vi "Inverted Pendulum Simulation.vi"() -> ()   [LabVIEW 2018]
uses:
  <vilib>/Simulation/Scripting/Companion Diagram/SimConfigNode/SimParams.ctl
  <vilib>/Simulation/Scripting/Companion Diagram/SimConfigNode/_simSolvers.ctl
  <vilib>/Simulation/Implementation/Shared/SIMSCR Execution Mode.ctl
  <vilib>/Platform/TimedLoop/XDataNode/timing_clust.ctl
  <vilib>/Platform/TimedLoop/XDataNode/nitl_modes.ctl
  <vilib>/Platform/TimedLoop/XDataNode/wakeup.ctl
  <vilib>/Simulation/Param Hierarchy/Typedefs/SIMPH Param Control Actions.ctl
  <vilib>/Simulation/Implementation/Shared/NILVSim_ParamChanged.vi
  <vilib>/Simulation/Implementation/Shared/NILVSim_FinishedLate.vi
  <vilib>/Simulation/Implementation/Shared/NILVSIM_BeginStep.vi
  <vilib>/Simulation/DataSources/Implementation/NILVSim Signal Generator.llb/SIM Signal Generator (scalar).vi
  <vilib>/Simulation/SignalDisplay/Implementation/NILVSim Time Waveform.llb/SIM Time Waveform (scalar).vi
  <vilib>/Simulation/SignalArithmetic/Implementation/NILVSim Gain.llb/SIM Gain (scalar).vi
  <vilib>/Simulation/Utility/Implementation/SIM Halt.vi
  <vilib>/Simulation/ContinuousLinear/Implementation/NILVSim State Space.llb/SIM State Space Distributor (CD).vi
  <vilib>/Simulation/SignalArithmetic/Implementation/NILVSim Gain.llb/SIM Gain (vector,ScalarGain).vi
  <vilib>/Simulation/SignalDisplay/Implementation/NILVSim Time Waveform.llb/SIM Time Waveform (vector).vi
  <vilib>/Simulation/SignalArithmetic/Implementation/NILVSim Gain.llb/SIM Gain (vector,MatrixGain).vi
  <vilib>/Simulation/ContinuousLinear/Implementation/NILVSim State Space.llb/SIM State Space Collector (CD).vi
  <vilib>/Simulation/Implementation/Shared/NILVSim_Manager.vi
  <vilib>/Utility/error.llb/Clear Errors.vi
  <vilib>/Simulation/Implementation/Shared/NILVSim_FinalizeModel.vi
  <vilib>/imath/engines/lvmath2/RunTimeEngine/IndexRead/NIMS M(S,S).vi
  <instcachedir>/0/NIMS M(S,S)_AC51E74150A542F7991B9634C66F3096.lvgen/NIMS M(S,S)_AC51E74150A542F7991B9634C66F3096_000.vi
  <vilib>/imath/engines/lvmath2/RunTimeEngine/IndexRead/NIMS V(S).vi
  <instcachedir>/0/NIMS V(S)_0488751826AF41519A22953C041130DC.lvgen/NIMS V(S)_0488751826AF41519A22953C041130DC_000.vi
  <vilib>/imath/engines/lvmath2/RunTimeEngine/IndexReplace/NIMS M(S,S)=S.vi
  <instcachedir>/0/NIMS M(S,S)=S_5DAF17B45D8A4C8588C7CF468644990A.lvgen/NIMS M(S,S)=S_5DAF17B45D8A4C8588C7CF468644990A_000.vi
  <vilib>/imath/engines/lvmath2/RunTimeEngine/ErrorHandling/NIMS_Create Error From Enums.vi
  <vilib>/imath/engines/lvmath/Plug In/Control Design/BuiltInFunctions/ss/NIMS_CD_ss(A,B,C,D).vi
  <vilib>/imath/engines/lvmath2/RunTimeEngine/NodeEndStatement/NIMS_NodeEndStatement_Output.vi
  <instcachedir>/0/NIMS_NodeEndStatement_Output_53EC0D466D134D7ABD903AC30B43404B.lvgen/NIMS_NodeEndStatement_Output_53EC0D466D134D7ABD903AC30B43404B_011.vi
  <vilib>/imath/engines/lvmath2/RunTimeEngine/ErrorHandling/NIMS_Finalize Error.vi
  <vilib>/Simulation/Implementation/Shared/SIM Unbundle Sim Info.vi
  <vilib>/Simulation/Implementation/Shared/SIMSH Read Queue.vi
  <vilib>/Simulation/Implementation/Shared/NILVSim_Initialize.vi
  <vilib>/Simulation/Utility/Implementation/NILVSim Get Time and IsAcceptedStep.vi
  <vilib>/Simulation/Implementation/Shared/NILVSim_GetModelError.vi
  <vilib>/Simulation/Implementation/Shared/SIM Bundle Sim Info.vi
  <vilib>/Simulation/Scripting/Companion Diagram/SimConfigNode/SimDog.xnode
  <vilib>/addons/Control Design/_Model Construction/Model Typedefs.llb/CD State Space Model (MIMO).ctl
  <vilib>/addons/Control Design/_Model Construction/Model Typedefs.llb/CD General Elements.ctl
  <vilib>/Platform/TimedLoop/XDataNode/XDataNode.xnode
  <vilib>/Simulation/Implementation/XNodeFramework/SimXNode/SimX.xnode
  <vilib>/addons/Control Design/_Model Construction/NI_LinSys_Model Typedefs.lvlib
  <vilib>/Simulation/ContinuousLinear/Implementation/NILVSim State Space.llb/SIM State Space (CD).vi
  <vilib>/Platform/TimedLoop/XDataNode/XDNodeRunTimeDep.lvlib
  <vilib>/Simulation/Implementation/Shared/NI_SIM_Implementation.lvlib
panel:
  out "Reference":waveform(dbl)(graph)
  in  "Feedback Gain":dbl[][](array[numeric])
  out "Output":waveform(dbl)[](graph)=[{"t0"=timestamp(14.86 s since 1904-01-01), "dt"=1.0, "Y"=[20.0]}, {"t0"=timestamp(14.86 s since 1904-01-01), "dt"=1.0, "Y"=[19.893873916201358]}]
  out "State":waveform(dbl)[](graph)=[{"t0"=timestamp(14.86 s since 1904-01-01), "dt"=1.0, "Y"=[20.0]}, {"t0"=timestamp(14.86 s since 1904-01-01), "dt"=1.0, "Y"=[19.893873916201358]}]
  in  "Frequency (Hz)":dbl(slide)=0.2 min=0.0 max=0.5 step=0.05 scale=0.0..0.5 scale format="%#_3f"
  in  "Amplitude (deg)":dbl(slide)=20.0 min=0.0 max=40.0 step=5.0 scale=0.0..40.0
  in  "stop":bool
  # "Rotary Arm Reference Signal"
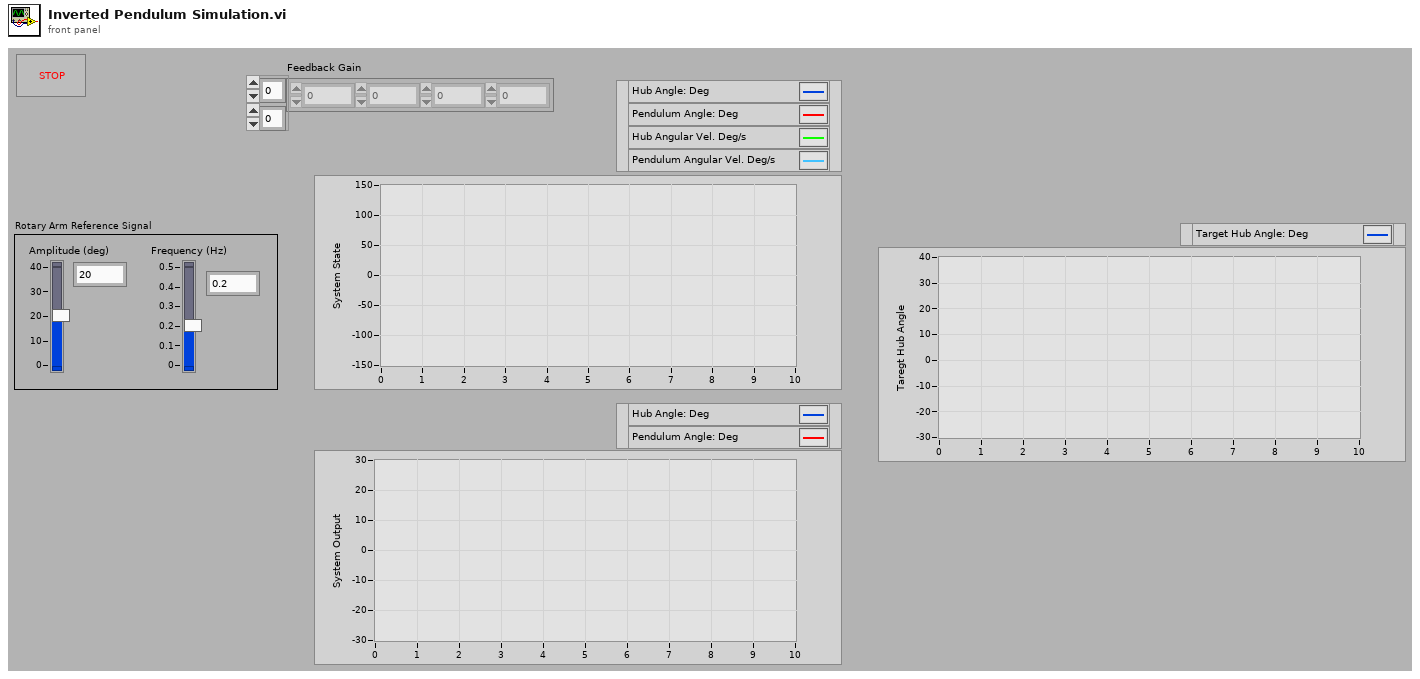
[diagram p1: front panel]
types:
  T1 = typedef "NI_LinSys_Model Typedefs.lvlib/CD State Space Model (MIMO).ctl" = cluster{"properties":T2, "A":dbl[][], "B":dbl[][], "C":dbl[][], "D":dbl[][], "StateNames":string[], "Transport Delay":dbl[][]}
  T2 = typedef "NI_LinSys_Model Typedefs.lvlib/CD General Elements.ctl" = cluster{"Model name":string, "Input names":string[], "Output names":string[], "Input Delays":dbl[], "Output Delays":dbl[], "Sampling Time":dbl, "Notes":string}
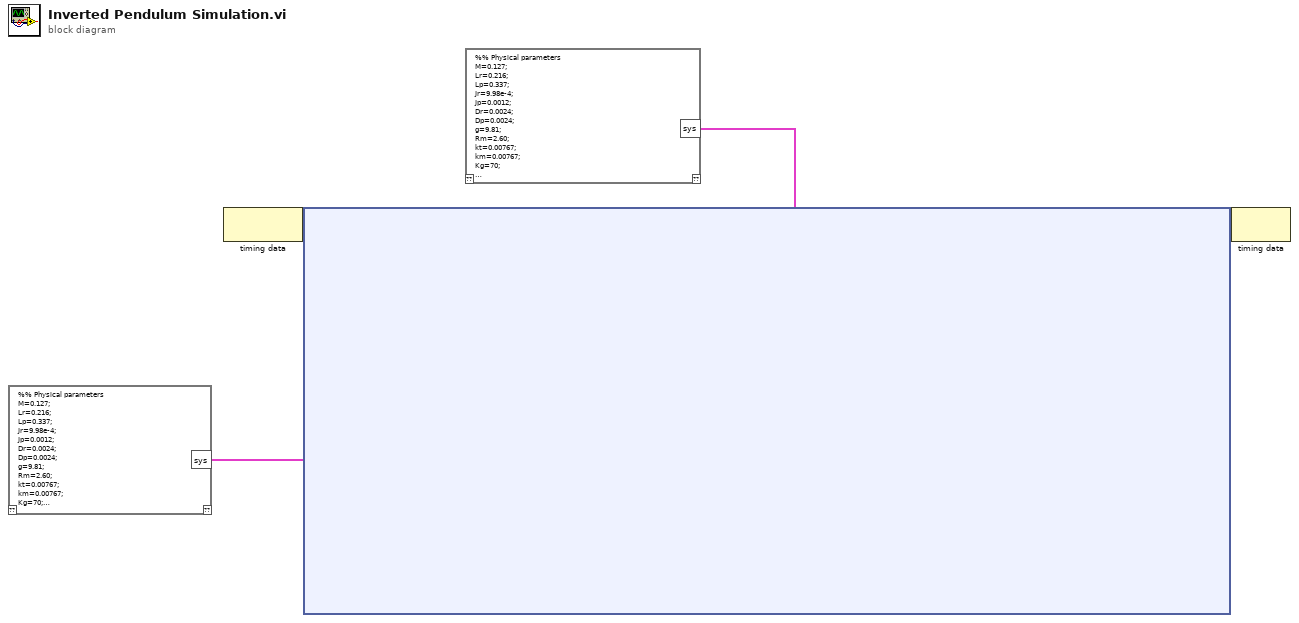
[diagram p0: block diagram]
diagram:
  n1 = mathscript code="%% Physical parameters\nM=0.127;\nLr=0.216;\nLp=0.337;\nJr=9.98e-4;\nJp=0.0012;\nDr=0.0024;\nDp=0.0024;\ng=9.81;\nRm=2.60;\nkt=0.00767;\nkm=0.00767;\nKg=70;\n\nJt = Jr*Jp + M*(Lp/2)^2*Jr + Jp*M*Lr^2;\nA = [0 0 1 0;\n         0 0 0 1;\n         0 M^2*(Lp/2)^2*Lr*g/Jt -Dr*(Jp+M*(Lp/2)^2)/Jt -M*(Lp/2)*Lr*Dp/Jt;\n         0 M*g*(Lp/2)*(Jr+M*Lr^2)/Jt -M*(Lp/2)*Lr*Dr/Jt -Dp*(Jr+M*Lr^2)/Jt];\n\nB = [0; 0; (Jp+M*(Lp/2)^2)/Jt; M*(Lp/2)*Lr/Jt];\nC = eye(2,4);\nD = zeros(2,1);\n\n% Add actuator dynamics\nA(3,3) = A(3,3) - Kg^2*kt*km/Rm*B(3);\nA(4,3) = A(4,3) - Kg^2*kt*km/Rm*B(4);\nB = Kg * kt * B / Rm;\n\nsys=ss(A,B,C,D);"() -> ("sys"=w1:T1)  [unwired: 1 in, 1 out]
  n2 = node-c288() -> (w4:variant)  [unwired: 1 in]
  n3 = mathscript code="%% Physical parameters\nM=0.127;\nLr=0.216;\nLp=0.337;\nJr=9.98e-4;\nJp=0.0012;\nDr=0.0024;\nDp=0.0024;\ng=9.81;\nRm=2.60;\nkt=0.00767;\nkm=0.00767;\nKg=70;\n\nJt = Jr*Jp + M*(Lp/2)^2*Jr + Jp*M*Lr^2;\nA = [0 0 1 0;\n         0 0 0 1;\n         0 M^2*(Lp/2)^2*Lr*g/Jt -Dr*(Jp+M*(Lp/2)^2)/Jt -M*(Lp/2)*Lr*Dp/Jt;\n         0 M*g*(Lp/2)*(Jr+M*Lr^2)/Jt -M*(Lp/2)*Lr*Dr/Jt -Dp*(Jr+M*Lr^2)/Jt];\n\nB = [0; 0; (Jp+M*(Lp/2)^2)/Jt; M*(Lp/2)*Lr/Jt];\nC = eye(2,4);\nD = zeros(2,1);\n\n% Add actuator dynamics\n\nA(3,3) = A(3,3) - Kg^2*kt*km/Rm*B(3);\nA(4,3) = A(4,3) - Kg^2*kt*km/Rm*B(4);\nB = Kg * kt * B / Rm;\n\nsys=ss(A,B,C,D);"() -> ("sys"=w2:T1)  [unwired: 1 in, 1 out]
  n4 = node-c254 ("Control & Simulation Loop")(w4, w2, w1) -> (w3:variant)
  n5 = node-c288(w3) -> ()  [unwired: 1 out]
